vi "N6701A_Open.vi"(8 "error in (no error)":errorcluster, 9 "Open Session":bool, 10 "Reset Instr":bool, 11 "VISA Name":refnum<visa-resource-name>) -> (0 "error out":errorcluster, 3 "Instrument handle":refnum<visa-resource-name>)   [LabVIEW 2015]
uses:
  <instrlib>/Agilent N6700 Series/Agilent N6700 Series.lvlib
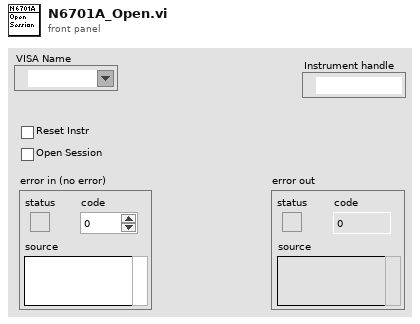
[diagram p1: front panel]
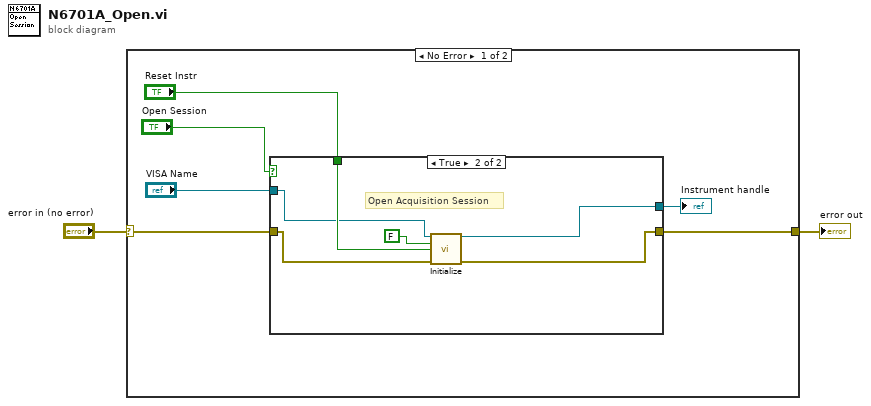
[diagram p0: block diagram]
diagram:
  n1 = case shown="No Error" "error in (no error)" {
    selector: "error in (no error)" -> [w5 w17]
    tunnel: [w4 w17] -> w1
    frame No Error {
      n2 = case shown="True" "Open Session" {
        tunnel: "VISA Name" -> [w9 w13]
        tunnel: "Reset Instr" -> [_ w16]
        tunnel: w5 -> [w10 w15]
        tunnel: [w10 w12] -> w4
        tunnel: [w9 w11] -> w3
        frame False {
        }
        frame True {
          # "Open Acquisition Session"
          n3 = call <instrlib>:"Initialize.vi"("VISA resource name"=w13, "ID Query? (T: Yes)"=FALSE ("ID Query"), "Reset? (T: Yes)"=w16, "error in (no error)"=w15) -> ("VISA resource name out"=w11:refnum<visa-resource-name>, "error out"=w12:errorcluster)  [unwired: 10 in]
        }
      }
      "Instrument handle" <- w3
    }
    frame Error {
    }
  }
  "error out" <- w1
